vi "HeaderDecoder.vi"(11 "input class":refnum<class "Text File.lvclass">) -> (3 "output class":refnum<class "Text File.lvclass">)   [LabVIEW 2020, in "Text File.lvclass"]
uses:
  Text File.lvclass
  Text File.lvclass/Text File.ctl
  Waveform Obj/Waveform Obj.lvclass/Waveform Obj.ctl
  Accessors/Read Text_ic type.vi
  Accessors/Read Text_Header.vi
  Waveform Obj/Accessors/Write play mode.vi
  Accessors/Write voltage idx.vi
  Waveform Obj/Accessors/Write wait.vi
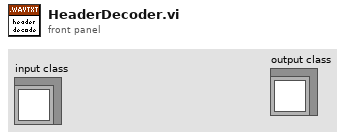
[diagram p1: front panel]
types:
  T1 = typedef "Haptic IC.lvclass/(Ctrl)IC Type.ctl" = enum8{"DW7800", "DW7802", "DW7912", "DW7914"}
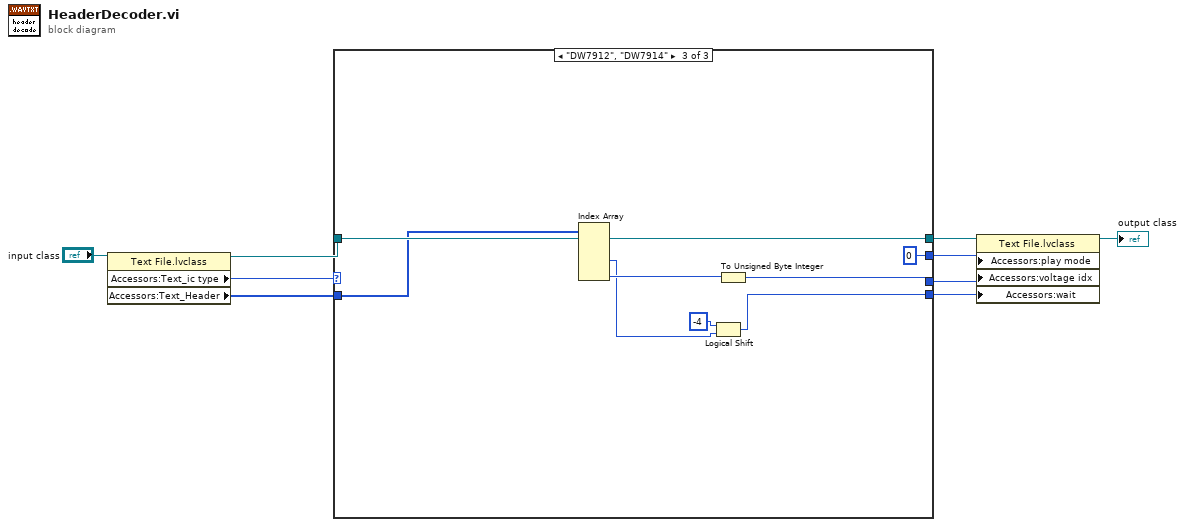
[diagram p0: block diagram]
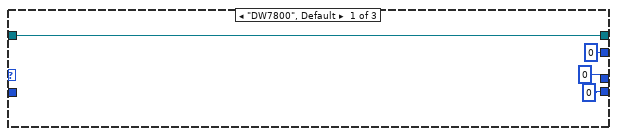
[diagram p2: hidden frame]
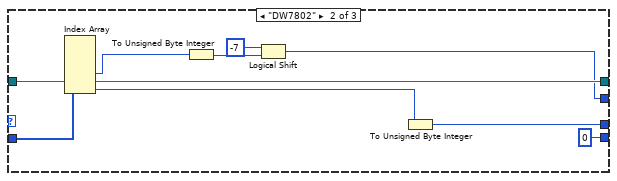
[diagram p3: hidden frame]
diagram:
  n1 = property class="Text File.lvclass"(reference="input class") -> (reference out=w4:refnum<class "Text File.lvclass">, "Accessors:Text_ic type"=w3:T1, "Accessors:Text_Header"=w2:u16[])  [unwired: 1 in, 1 out]
  n2 = case shown="\"DW7912\", \"DW7914\"" w3 {
    tunnel: w4 -> [w13 w22 w30]
    tunnel: [w13 w22 w30] -> w9
    tunnel: [u8 0 ("wait") u8 0 ("wait") w26] -> w7
    tunnel: [u8 0 ("play mode") w16 u8 0 ("play mode")] -> w6
    tunnel: w2 -> [_ w21 w29]
    tunnel: [u8 0 w14 w24] -> w1
    frame "DW7800", Default {
    }
    frame "DW7802" {
      n3 = Index Array(array=w21) -> (element #3=w19:u16, element #5=w15:u16)  [unwired: 5 in, 3 out]
      n4 = To Unsigned Byte Integer(number=w19) -> (unsigned 8bit integer=w17:u8)
      n5 = Logical Shift(y=i16 -7, x=w17) -> (x << y=w16:u8)
      n6 = To Unsigned Byte Integer(number=w15) -> (unsigned 8bit integer=w14:u8)
    }
    frame "DW7912", "DW7914" {
      n7 = Index Array(array=w29) -> (element #3=w23:u16, element #5=w25:u16)  [unwired: 5 in, 3 out]
      n8 = Logical Shift(y=i16 -4, x=w23) -> (x << y=w26:u16)
      n9 = To Unsigned Byte Integer(number=w25) -> (unsigned 8bit integer=w24:u8)
    }
  }
  n10 = property class="Text File.lvclass"(reference=w9, "Accessors:play mode"=w6, "Accessors:voltage idx"=w1, "Accessors:wait"=w7) -> (reference out=→"output class":refnum<class "Text File.lvclass">)  [unwired: 1 in, 1 out]
